vi "ReadTextFile.vi"(9 "file (use dialog)":path) -> (2 "String":string, 3 "Double":dbl)   [LabVIEW 2014]
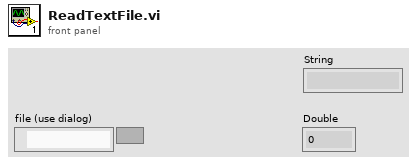
[diagram p1: front panel]
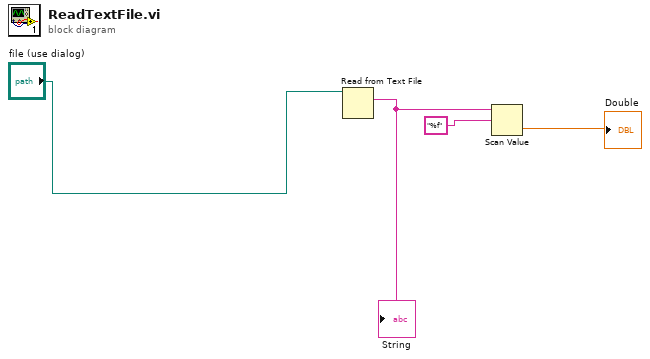
[diagram p0: block diagram]
diagram:
  n1 = Read from Text File(file (use dialog)="file (use dialog)") -> (text=w3:string)  [unwired: 3 in, 3 out]
  "String" <- w3
  n2 = Scan Value(string=w3, format string="%f") -> (value=→"Double":dbl)  [unwired: 1 in, 1 out]
